vi "19.7-Classicl IIR Filters.vi"() -> ()   [LabVIEW 2020]
doc: "Displays the Transfer Function of the filter selected from the front panel controls. \n\nYou can select any of the 5 IIR filter design methods (Bessel, Butterworth, Chebyshev I and II, and Elliptic) and the passband type (lowpass, highpass, bandpass, and bandstop)."
uses:
  <vilib>/Analysis/3filter.llb/Filter Passband Type.ctl
  <vilib>/Analysis/3filter.llb/Filter Frequence Specification (Design).ctl
  <vilib>/Analysis/3filter.llb/Filter Ripple Specification (Design).ctl
  <vilib>/Utility/error.llb/DialogType.ctl
  <vilib>/Analysis/baseanly.llb/IIR Cascade Filter (DBL).vi
  <vilib>/Analysis/NI_AALPro.lvlib
  <vilib>/Analysis/NI_AALBase.lvlib
  <vilib>/Analysis/NI_AAL_Filter.lvlib
panel:
  out "Filtered":dbl[](graph)
  out "Phase":cluster{dbl, dbl, dbl[]}(graph)
  out "Mag":cluster{dbl, dbl, dbl[]}(graph)
  out "Sig":dbl[](graph)
  out "Order":i32
  in  "Ripples":T1={"passband"=0.1, "stopband"=60.0, "dB/linear? (T: dB)"=TRUE}
  in  "Freq.":T2={"lower pass freq"=100.0, "lower stop freq"=260.0, "higher pass freq"=300.0, "higher stop freq"=350.0}
  in  "filter type":T3
  out "Msg":string
  in  "Stop":bool
  in  "Fs":dbl=1024.0 format="%#.6g"
  in  "Filter Design":T4(ring)
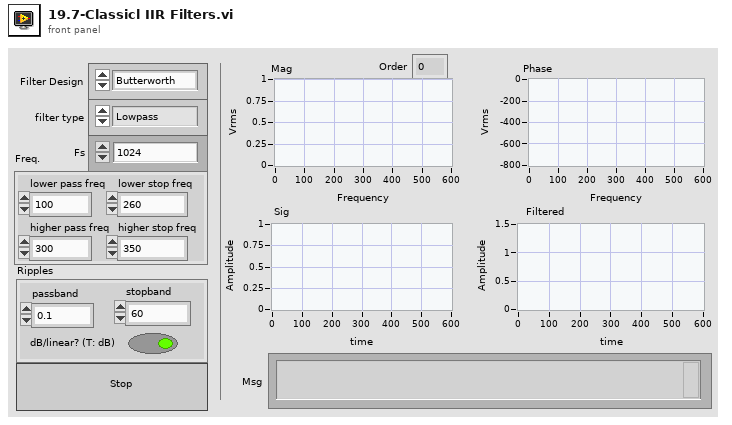
[diagram p1: front panel]
types:
  T1 = typedef "NI_AAL_Filter.lvlib/Filter Ripple Specification (Design).ctl" = cluster{"passband":dbl, "stopband":dbl, "dB/linear? (T: dB)":bool}
  T2 = typedef "NI_AAL_Filter.lvlib/Filter Frequence Specification (Design).ctl" = cluster{"lower pass freq":dbl, "lower stop freq":dbl, "higher pass freq":dbl, "higher stop freq":dbl}
  T3 = typedef "NI_AALBase.lvlib/Filter Passband Type.ctl" = enum32{"Lowpass", "Highpass", "Bandpass", "Bandstop"}
  T4 = enum16{"Butterworth", "Chebyshev", "Inverse Chebyshev", "Elliptic", "Bessel"}
  T5 = enum32{"Vrms", "Vpk", "Vrms^2", "Vpk^2", "Vrms/rtHz", "Vpk/rtHz", "Vrms^2/Hz", "Vpk^2/Hz"}
  T6 = enum16{"Power (Vrms^2)", "Amplitude (Vrms)", "Gain (amplitude ratio)"}
  T7 = typedef "DialogType.ctl" = u16
  T8 = cluster{"filter structure":enum32{"IIR 2nd Order", "IIR 4th Order"}, "Reverse Coefficients":dbl[], "Forward Coefficients":dbl[]}
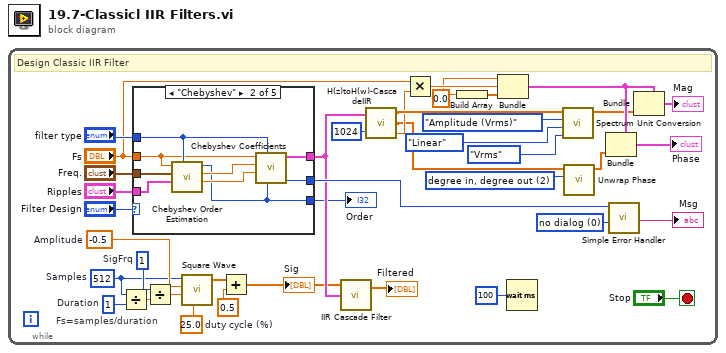
[diagram p0: block diagram]
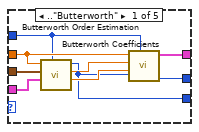
[diagram p2: hidden frame]
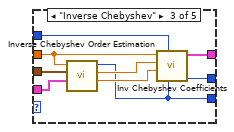
[diagram p3: hidden frame]
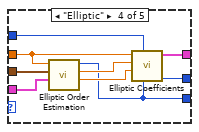
[diagram p4: hidden frame]
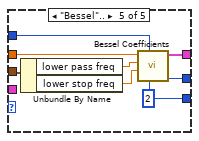
[diagram p5: hidden frame]
diagram:
  n1 = while {
    stop <- "Stop" stop-if-true
    w6 = 1  # Duration
    w12 = 1  # SigFrq
    w13 = 25.0  # duty cycle (%)
    w14 = -0.5  # Amplitude
    w8 = 512  # Samples
    w24 = 0.0
    w26 = T7 0 items=["no dialog", "OK message", "continue or stop message", "OK message + warnings", "continue/stop + warnings"] ("type of dialog (OK msg:1)")
    w31 = 2 items=["radian in, radian out", "radian in, degree out", "degree in, degree out", "degree in, radian out"] ("phase unit")
    # "Fs=samples/duration"
    # "Design Classic IIR Filter"
    n2 = Divide(x=w8, y=w6) -> (x/y=w7:dbl)
    n3 = case shown="\"Chebyshev\"" "Filter Design" {
      tunnel: "filter type" -> [w45 w53 w66 w75 w81]
      tunnel: "Fs" -> [w46 w52 w61 w72 w80]
      tunnel: [w48 w57 w65 w74 w83] -> w19
      tunnel: [w47 w56 w64 w73 w82] -> w25
      tunnel: "Freq." -> [w44 w55 w63 w71 w79]
      tunnel: "Ripples" -> [w43 w54 w62 w70 _]
      tunnel: [w40 w49 w58 w67 w76] -> w1
      frame .."Butterworth" {
        n4 = call <vilib>:"Butterworth Order Estimation.vi"("filter type"=w45, "ripple specs"=w43, "freq specs"=w44, "sampling freq: fs"=w46) -> ("low cutoff freq"=w41:dbl, "high cutoff freq"=w42:dbl, "estimated order"=w40:i32)  [unwired: 4 in, 1 out]
        n5 = call <vilib>:"Butterworth Coefficients.vi"("order"=w40, "filter type"=w45, "low cutoff freq: fl"=w41, "high cutoff freq: fh"=w42, "sampling freq: fs"=w46) -> ("error"=w47:i32, "IIR Filter Cluster"=w48:T8)  [unwired: 5 in]
      }
      frame "Chebyshev" {
        n6 = call <vilib>:"Chebyshev Order Estimation.vi"("filter type"=w53, "ripple specs"=w54, "freq specs"=w55, "sampling freq: fs"=w52) -> ("low cutoff freq"=w50:dbl, "high cutoff freq"=w51:dbl, "estimated order"=w49:i32)  [unwired: 3 in, 2 out]
        n7 = call <vilib>:"Chebyshev Coefficients.vi"("order"=w49, "filter type"=w53, "low cutoff freq: fl"=w50, "high cutoff freq: fh"=w51, "sampling freq: fs"=w52) -> ("error"=w56:i32, "IIR Filter Cluster"=w57:T8)  [unwired: 5 in]
      }
      frame "Inverse Chebyshev" {
        n8 = call <vilib>:"Inverse Chebyshev Order Estimation.vi"("ripple specs"=w62, "freq specs"=w63, "sampling freq: fs"=w61) -> ("low cutoff freq"=w59:dbl, "high cutoff freq"=w60:dbl, "estimated order"=w58:i32)  [unwired: 4 in, 2 out]
        n9 = call <vilib>:"Inv Chebyshev Coefficients.vi"("order"=w58, "filter type"=w66, "low cutoff freq: fl"=w59, "high cutoff freq: fh"=w60, "sampling freq: fs"=w61) -> ("error"=w64:i32, "IIR Filter Cluster"=w65:T8)  [unwired: 5 in]
      }
      frame "Elliptic" {
        n10 = call <vilib>:"Elliptic Order Estimation.vi"("ripple specs"=w70, "freq specs"=w71, "sampling freq: fs"=w72) -> ("low cutoff freq"=w68:dbl, "high cutoff freq"=w69:dbl, "estimated order"=w67:i32)  [unwired: 4 in, 2 out]
        n11 = call <vilib>:"Elliptic Coefficients.vi"("order"=w67, "filter type"=w75, "low cutoff freq: fl"=w68, "high cutoff freq: fh"=w69, "sampling freq: fs"=w72) -> ("error"=w73:i32, "IIR Filter Cluster"=w74:T8)  [unwired: 5 in]
      }
      frame "Bessel".. {
        w76 = 2 ("order")
        n12 = Unbundle By Name(w79) -> ("lower pass freq"=w78:dbl, "lower stop freq"=w77:dbl)
        n13 = call <vilib>:"Bessel Coefficients.vi"("order"=w76, "filter type"=w81, "low cutoff freq: fl"=w77, "high cutoff freq: fh"=w78, "sampling freq: fs"=w80) -> ("error"=w82:i32, "IIR Filter Cluster"=w83:T8)  [unwired: 5 in]
      }
    }
    "Order" <- w1
    n14 = Divide(x=w12, y=w7) -> (x/y=w9:dbl)
    n15 = call <vilib>:"Square Wave.vi"("samples"=w8, "amplitude"=w14, "frequency"=w9, "duty cycle (%)"=w13) -> ("square wave"=w11:dbl[])  [unwired: 2 in, 2 out]
    n16 = Add(x=w11, y=0.5) -> (x+y=w4:dbl[])
    "Sig" <- w4
    n17 = call-poly <vilib>:"IIR Cascade Filter.vi"("IIR Filter Cluster"=w19, "X"=w4) -> ("Filtered X"=→"Filtered":dbl[])  [unwired: 1 in, 1 out]
    n18 = call "H(z)toH(w)-CascadeIIR.vi"("IIR Filter Cluster"=w19, "FFT size"=1024) -> ("Mag H(w)"=w18:dbl[], "Phase H(w)"=w16:dbl[], "df"=w17:dbl)
    n19 = Multiply(x="Fs", y=w17) -> (x*y=w37:dbl)
    n20 = Build Array ("array")(w24) -> (w36:dbl[])
    n21 = Bundle(w24, w37, w36) -> (w39:cluster{dbl, dbl, dbl[]})  [unwired: 1 in]
    n22 = Wait (ms)(milliseconds to wait=u32 100) -> ()  [unwired: 1 out]
    n23 = call <vilib>:"Spectrum Unit Conversion.vi"("display unit"=T5."Vrms", "log/linear"=enum16{"Linear", "dB", "dBm"}."Linear", "spectrum type"=T6."Amplitude (Vrms)", "Spectrum in"=w18) -> ("Spectrum out"=w32:dbl[])  [unwired: 6 in, 1 out]
    n24 = call <vilib>:"Unwrap Phase.vi"("phase unit"=w31, "Phase"=w16) -> ("Unwrapped Phase"=w38:dbl[])  [unwired: 8 in, 1 out]
    n25 = Bundle(cluster=w39, w38) -> (→"Phase":cluster{dbl, dbl, dbl[]})  [unwired: 2 in]
    n26 = call <vilib>:"Simple Error Handler.vi"("error code (no error:0)"=w25, "type of dialog (OK msg:1)"=w26) -> ("message"=→"Msg":string)  [unwired: 3 in, 4 out]
    n27 = Bundle(cluster=w39, w32) -> (→"Mag":cluster{dbl, dbl, dbl[]})  [unwired: 2 in]
  }
